vi "ConvertDLPVAGainIndex.vi"(1 "Numeric 2":i16) -> (0 "Numeric":dbl)   [LabVIEW 2013]
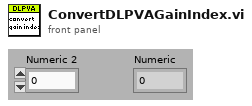
[diagram p1: front panel]
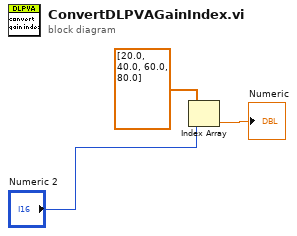
[diagram p0: block diagram]
diagram:
  n1 = Index Array(array=dbl[] [20.0, 40.0, 60.0, 80.0], index="Numeric 2") -> (element=→"Numeric":dbl)
